vi "Uploading to ELVIS Global Variables.vi"() -> ()   [LabVIEW 2019]
doc: "Global variables for transfering data between VIs while the Uploading Audio File is running."
panel:
  in  "Message Color":u32(colorbox)
  out "Message":string
  out "Audio Signal Out":dbl(graph) caption="data file"
  # "Global variables for transfering data while the subVI is in progress."
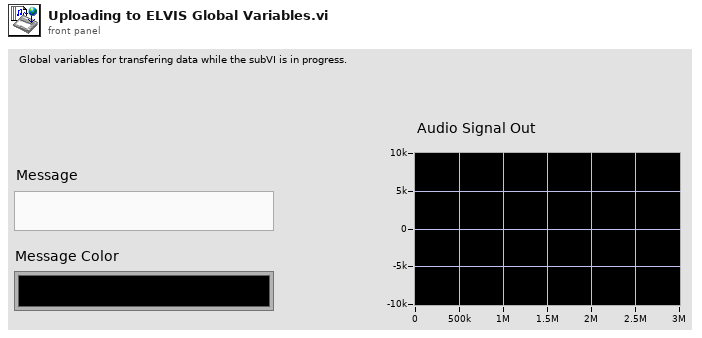
[diagram p1: front panel]
diagram:
